vi "Reference pressure module - Get P.vi"() -> ()   [LabVIEW 2020]
uses:
  Arduino/ctls_and_globals/Arduino tx msg cluster.ctl
panel:
  out "Scan comment":string
  out "P (Pa)":dbl
  in  "Port":refnum<visa-resource-name>
  in  "Address":u8=1
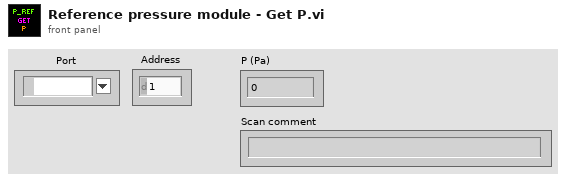
[diagram p1: front panel]
types:
  T1 = typedef "Arduino tx msg cluster.ctl" = cluster{"dest":u8, "A/D/C/I":string, "R/W":string, "chan":u8, "val (float)":sgl}
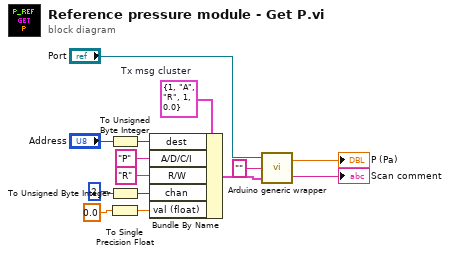
[diagram p0: block diagram]
diagram:
  w11 = T1 {"dest"=1, "A/D/C/I"="A", "R/W"="R", "chan"=1, "val (float)"=0.0}  # Tx msg cluster
  n1 = To Unsigned Byte Integer(number="Address") -> (unsigned 8bit integer=w9:u8)
  n2 = To Unsigned Byte Integer(number=u8 2) -> (unsigned 8bit integer=w10:u8)
  n3 = To Single Precision Float(number=0.0) -> (single precision float=w7:sgl)
  n4 = Bundle By Name(cluster=w11, "dest"=w9, "A/D/C/I"="P" ("A/D"), "R/W"="R", "chan"=w10, "val (float)"=w7) -> (w8:T1)
  n5 = call "Arduino generic wrapper.vi"("Tx msg cluster"=w8, "Channel Name"="", "Port name"="Port") -> ("Scan comment"=→"Scan comment":string, "Output"=→"P (Pa)":dbl)
